vi "Untitled 3.vi"() -> ()   [LabVIEW 2018, in "Sensor Dispense.lvclass"]
uses:
  Sensor Dispense.lvclass
  C:/Users/HEP/Documents/GitHub/New folder/C/Users/HEP/Documents/GitHub/UCSB-Gantry-HEP-2018/Classes/Routine/Dispense/Dispense.lvclass
panel:
  out "Coordinates.CAD Cluster":T1(array[cluster])
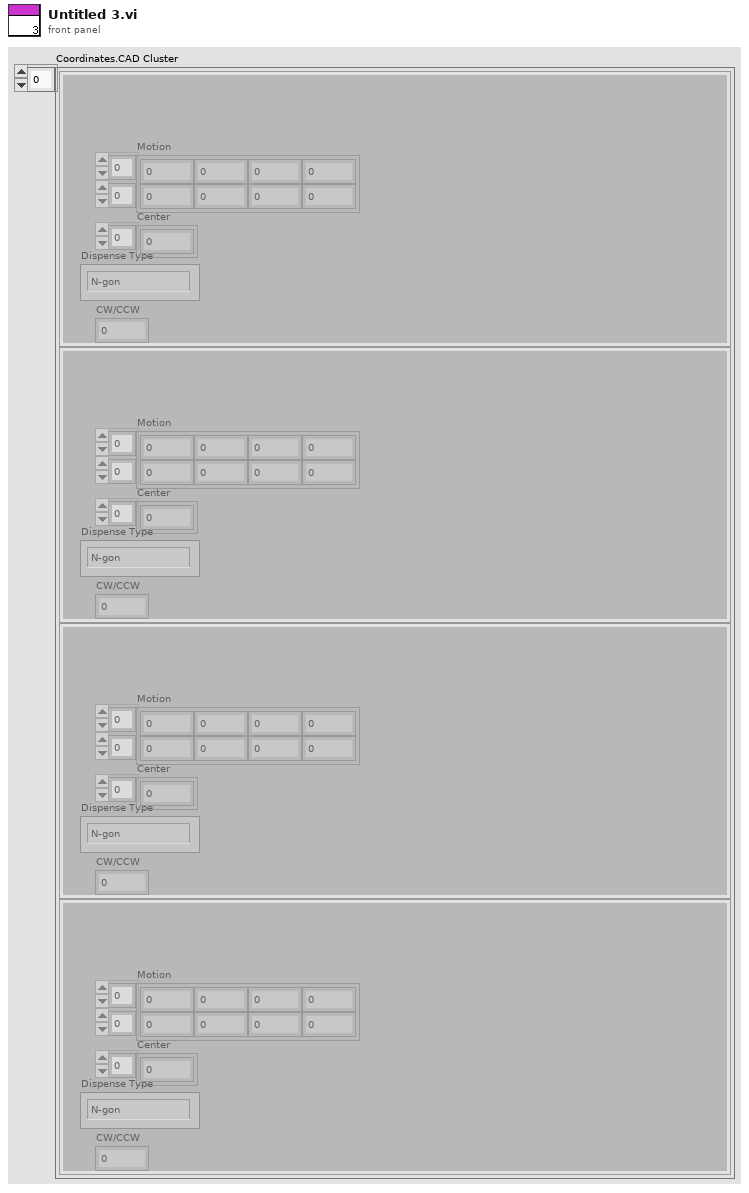
[diagram p1: front panel]
types:
  T1 = cluster{"Motion":dbl[][], "Center":dbl[], "CW/CCW":dbl, "Dispense Type":enum16{"N-gon", "Square", "Arc", "Dot", "Line", "Circle"}}[]
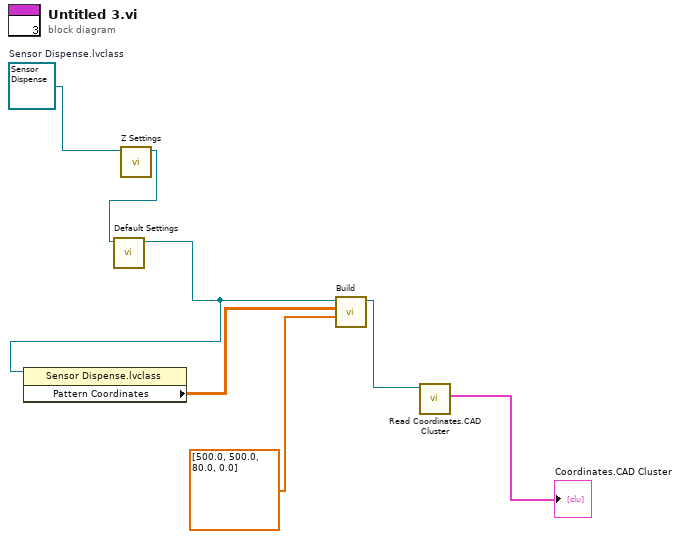
[diagram p0: block diagram]
diagram:
  w2 = refnum<class "Sensor Dispense.lvclass"> refnum  # Sensor Dispense.lvclass
  n1 = call-dynamic "Z Settings.vi"("Dispense in"=w2) -> ("Dispense out"=w1:refnum<class "Sensor Dispense.lvclass">)  [unwired: 9 in, 1 out]
  n2 = call-dynamic "Default Settings.vi"("Sensor Dispense in"=w1) -> ("Sensor Dispense out"=w6:refnum<class "Sensor Dispense.lvclass">)  [unwired: 9 in, 1 out]
  n3 = property class="Sensor Dispense.lvclass"(reference=w6) -> ("Pattern Coordinates"=w5:dbl[][])  [unwired: 1 in, 2 out]
  n4 = call-dynamic "Build.vi"("XYZTheta"=dbl[] [500.0, 500.0, 80.0, 0.0], "text file"=w5, "Sensor Dispense in"=w6) -> ("Sensor Dispense out"=w4:refnum<class "Sensor Dispense.lvclass">)  [unwired: 8 in]
  n5 = call-dynamic "Read Coordinates.CAD Cluster.vi"("Sensor Dispense in"=w4) -> ("Coordinates.CAD Cluster"=→"Coordinates.CAD Cluster":T1)  [unwired: 8 in, 2 out]
